vi "S2C_CMD_UpdateParameters.vi"(8 "Error In":errorcluster, 9 "Row":i32, 10 "CtlRef":refnum<vi>, 11 "ItemTag":string) -> (0 "Error Out":errorcluster)   [LabVIEW 2015]
doc: "Updates the command input parameter value after a popup menu selection."
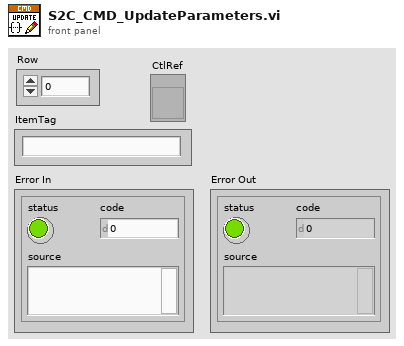
[diagram p1: front panel]
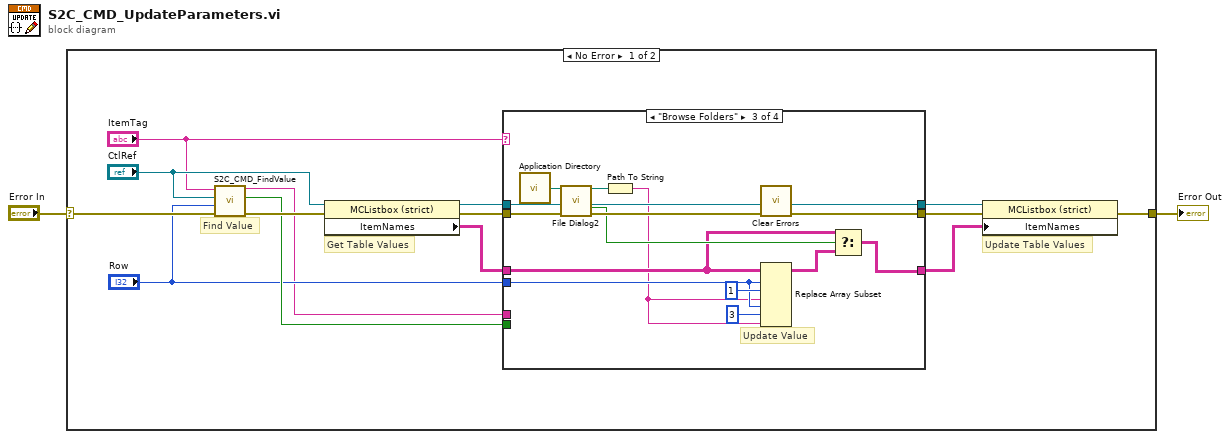
[diagram p0: block diagram]
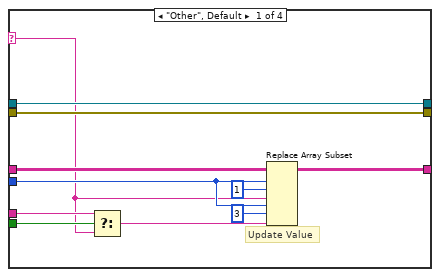
[diagram p2: hidden frame]
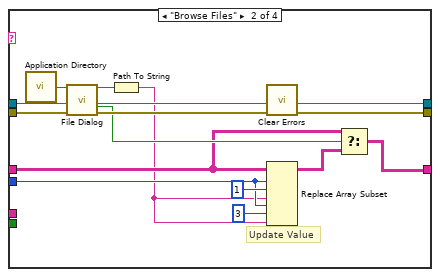
[diagram p3: hidden frame]
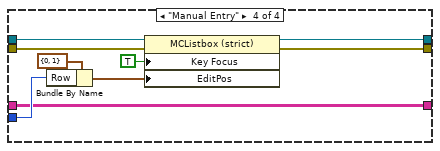
[diagram p4: hidden frame]
diagram:
  n1 = case shown="No Error" "Error In" {
    selector: "Error In" -> [w16 w65]
    tunnel: [w5 w65] -> w1
    frame No Error {
      # "Get Table Values"
      # "Update Table Values"
      # "Find Value"
      n2 = call "S2C_CMD_FindValue.vi"("Error In"=w16, "Row"="Row", "CtlRef"="CtlRef", "ItemTag"="ItemTag") -> ("Error Out"=w13:errorcluster, "Found?"=w12:bool, "Value_Int"=w10:string)  [unwired: 5 in]
      n3 = property on="Property Node" class="MCListbox (strict)"(reference="CtlRef", error in=w13) -> (reference out=w4:refnum<vi>, error out=w8:errorcluster, "ItemNames"=w14:string[][])
      n4 = case shown="\"Browse Folders\"" "ItemTag" {
        selector: "ItemTag" -> [w17 _ _ _]
        tunnel: [w24 w33 w47 w56] -> w15
        tunnel: w14 -> [w19 w35 w49 w56]
        tunnel: w12 -> [w23 _ _ _]
        tunnel: "Row" -> [w18 w31 w45 w57]
        tunnel: w10 -> [w22 _ _ _]
        tunnel: w8 -> [w21 w39 w53 w59]
        tunnel: [w21 w28 w42 w62] -> w7
        tunnel: w4 -> [w20 w32 w46 w58]
        tunnel: [w20 w32 w46 w63] -> w3
        frame "Other", Default {
          # "Update Value"
          n5 = Select(t=w22, s=w23, f=w17) -> (s? t:f=w27:string)
          n6 = Replace Array Subset(array=w19, new element #1=w17, index (row) #1=w18, index (col) #1=1 ("disabled index (col)"), new element #2=w27, index (row) #2=w18, index (col) #2=3 ("disabled index (col)")) -> (w24:string[][])
        }
        frame "Browse Files" {
          # "Update Value"
          n7 = call <vilib>:"Application Directory.vi"() -> ("Application Directory"=w40:path)
          n8 = call "File Dialog"("start path"=w40, "error in"=w39) -> ("selected path"=w38:path, "cancelled"=w36:bool, "error out"=w37:errorcluster)  [unwired: 10 in, 1 out]
          n9 = Path To String(path=w38) -> (string=w29:string)
          n10 = call <vilib>:"Clear Errors.vi"("error in (no error)"=w37) -> ("error out"=w28:errorcluster)  [unwired: 5 in, 1 out]
          n11 = Replace Array Subset(array=w35, new element #1=w29, index (row) #1=w31, index (col) #1=1 ("disabled index (col)"), new element #2=w29, index (row) #2=w31, index (col) #2=3 ("disabled index (col)")) -> (w34:string[][])
          n12 = Select(t=w35, s=w36, f=w34) -> (s? t:f=w33:string[][])
        }
        frame "Browse Folders" {
          # "Update Value"
          n13 = call <vilib>:"Application Directory.vi"() -> ("Application Directory"=w54:path)
          n14 = call "File Dialog2"("start path"=w54, "error in"=w53) -> ("selected path"=w52:path, "cancelled"=w50:bool, "error out"=w51:errorcluster)  [unwired: 10 in, 1 out]
          n15 = Path To String(path=w52) -> (string=w43:string)
          n16 = call <vilib>:"Clear Errors.vi"("error in (no error)"=w51) -> ("error out"=w42:errorcluster)  [unwired: 5 in, 1 out]
          n17 = Replace Array Subset(array=w49, new element #1=w43, index (row) #1=w45, index (col) #1=1 ("disabled index (col)"), new element #2=w43, index (row) #2=w45, index (col) #2=3 ("disabled index (col)")) -> (w48:string[][])
          n18 = Select(t=w49, s=w50, f=w48) -> (s? t:f=w47:string[][])
        }
        frame "Manual Entry" {
          n19 = Bundle By Name(cluster=cluster{"Row":i32, "Column":i32} {"Row"=0, "Column"=1} ("Edit Position"), "Row"=w57) -> (w61:cluster{"Row":i32, "Column":i32})
          n20 = property on="Property Node" class="MCListbox (strict)"(reference=w58, error in=w59, "Key Focus"=TRUE, "EditPos"=w61) -> (reference out=w63:refnum<vi>, error out=w62:errorcluster)
        }
      }
      n21 = property on="Property Node" class="MCListbox (strict)"(reference=w3, error in=w7, "ItemNames"=w15) -> (error out=w5:errorcluster)  [unwired: 1 out]
    }
    frame Error {
    }
  }
  "Error Out" <- w1
